vi "UI Refresh Data.vi"(8 "error in (no error)":errorcluster, 11 "GObject View in":refnum<class "VI List View.lvclass">) -> (0 "error out":errorcluster, 3 "GObject View out":refnum<class "VI List View.lvclass">)   [LabVIEW 2013, in "SET Project Editor.lvlib" / "VI List View.lvclass"]
uses:
  VI List View.lvclass
  VI List View.lvclass/VI List View.ctl
  UI View/UI View.lvclass/UI View.ctl
  SET Project Data/Project Data Class/Project Data.lvclass
  SET Project Data/VI Class/VI Data.lvclass
  UI View/Read _LangData.vi
  SET Project Data/Control Classes/GObject/GObject.lvclass
  SET Project Editor.lvlib
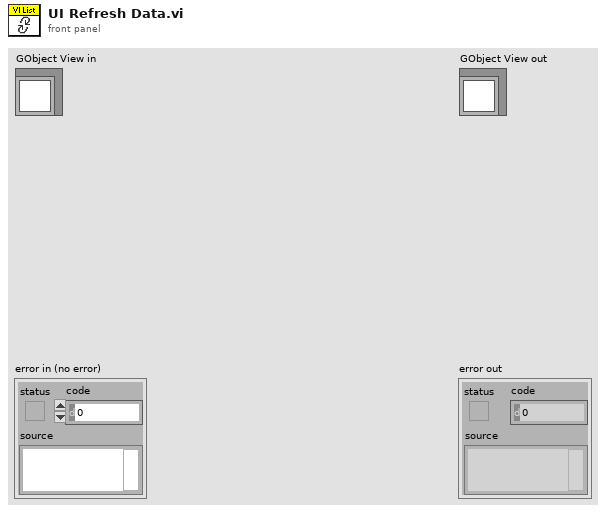
[diagram p1: front panel]
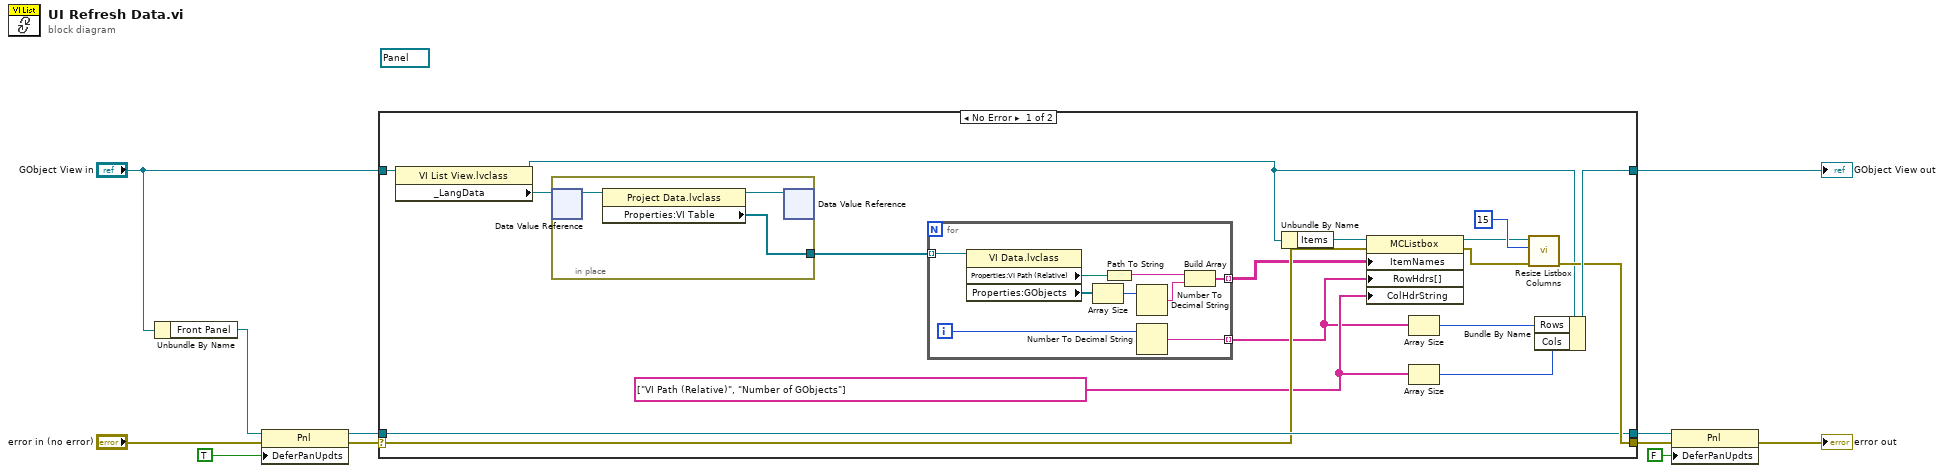
[diagram p0: block diagram]
diagram:
  (unwired) refnum<vi> refnum ("Front Panel")
  n1 = Unbundle By Name("GObject View in") -> ("Front Panel"=w9:refnum<vi>)
  n2 = property class="Pnl"(reference=w9, error in="error in (no error)", "DeferPanUpdts"=TRUE ("Defer Panel Updates")) -> (reference out=w5:refnum<vi>, error out=w6:errorcluster)
  n3 = case shown="No Error" w6 {
    selector: w6 -> [w19 w43]
    tunnel: [w24 w43] -> w3
    tunnel: [w28 w42] -> w11
    tunnel: "GObject View in" -> [w17 w42]
    tunnel: w5 -> [w21 w41]
    tunnel: [w21 w41] -> w4
    frame No Error {
      w18 = string[] ["VI Path (Relative)", "Number of GObjects"]
      n4 = property class="VI List View.lvclass"(reference=w17) -> (reference out=w12:refnum<class "VI List View.lvclass">, "_LangData"=w16:refnum<data-value>)  [unwired: 1 in, 1 out]
      n5 = in-place {
        in-place-border: [w29] -> w15
        n6 = in-place-dvr #1(w16) -> (w31:refnum<class "Project Data.lvclass">)  [unwired: 1 out]
        n7 = property class="Project Data.lvclass"(reference=w31) -> (reference out=w30:refnum<class "Project Data.lvclass">, "Properties:VI Table"=w29:refnum<class "VI Data.lvclass">[])  [unwired: 1 in, 1 out]
        n8 = in-place-dvr #1(w30) -> ()  [unwired: 2 out]
      }
      n9 = for {
        tunnel: w15 -> [w40] mode=indexing
        tunnel: [w34] -> w14 mode=indexing
        tunnel: [w32] -> w13 mode=indexing
        i -> [w33]
        n10 = property class="VI Data.lvclass"(reference=w40) -> ("Properties:VI Path (Relative)"=w39:path, "Properties:GObjects"=w37:refnum<class "GObject.lvclass">[])  [unwired: 1 in, 2 out]
        n11 = Array Size(array=w37) -> (size(s)=w38:i32)
        n12 = Path To String(path=w39) -> (string=w36:string)
        n13 = Number To Decimal String(number=w38) -> (decimal integer string=w35:string)  [unwired: 1 in]
        n14 = Number To Decimal String(number=w33) -> (decimal integer string=w32:string)  [unwired: 1 in]
        n15 = Build Array(w36, w35) -> (w34:string[])
      }
      n16 = Unbundle By Name(w12) -> ("Items"=w20:refnum<vi>)
      n17 = property class="MCListbox"(reference=w20, error in=w19, "ItemNames"=w14, "RowHdrs[]"=w13, "ColHdrString"=w18) -> (reference out=w26:refnum<vi>, error out=w25:errorcluster)
      n18 = Array Size(array=w13) -> (size(s)=w23:i32)
      n19 = Array Size(array=w18) -> (size(s)=w22:i32)
      n20 = call "Resize Listbox Columns.vi"("error in (no error)"=w25, "Padding (5px)"=i16 15, "Listbox Control ref in"=w26) -> ("error out"=w24:errorcluster)  [unwired: 7 in, 1 out]
      n21 = Bundle By Name(cluster=w12, "Rows"=w23, "Cols"=w22) -> (w28:refnum<class "VI List View.lvclass">)
    }
    frame Error {
    }
  }
  "GObject View out" <- w11
  n22 = property class="Pnl"(reference=w4, error in=w3, "DeferPanUpdts"=FALSE ("Defer Panel Updates")) -> (error out=→"error out":errorcluster)  [unwired: 1 out]
